vi "VI Tree.vi"   [LabVIEW 2025]
doc: "This is the instrument driver for the <INSTRUMENT NAME>. The VI Tree displays all the user-callable VIs of the instrument driver in an organized table."
panel:
  # "(c) 2025 RAMON TABOADA.  ALL RIGHTS RESERVED."
  # "SEE DIAGRAM\nFOR VI TREE."
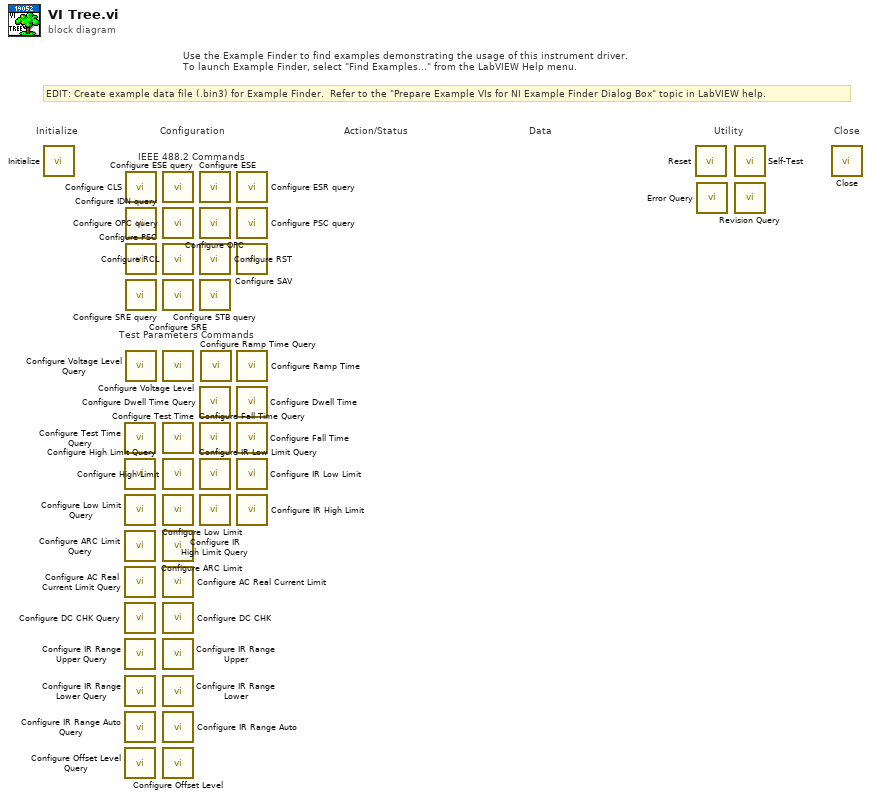
[diagram p0: block diagram]
diagram:
  # "Test Parameters Commands"
  # "IEEE 488.2 Commands"
  # "EDIT: Create example data file (.bin3) for Example Finder.  Refer to the \"Prepare Example VIs for NI Example Finder Dialog Box\" topic in LabVIEW help."
  # "Use the Example Finder to find examples demonstrating the usage of this instrument driver.\nTo launch Example Finder, select \"Find Examples...\" from the LabVIEW Help menu."
  # "Configuration"
  # "Utility"
  # "Data"
  # "Action/Status"
  # "Close"
  # "Initialize"
  n1 = call <instrlib>:"Initialize.vi"() -> ()  [unwired: 10 in, 2 out]
  n2 = call "Configure Test Time Query.vi"() -> ()  [unwired: 9 in, 3 out]
  n3 = call "Configure High Limit Query.vi"() -> ()  [unwired: 9 in, 3 out]
  n4 = call "Configure Low Limit Query.vi"() -> ()  [unwired: 9 in, 3 out]
  n5 = call "Configure ARC Limit Query.vi"() -> ()  [unwired: 9 in, 3 out]
  n6 = call "Configure AC Real Current Limit Query.vi"() -> ()  [unwired: 8 in, 3 out]
  n7 = call "Configure DC CHK Query.vi"() -> ()  [unwired: 10 in, 2 out]
  n8 = call "Configure IR Range Upper Query.vi"() -> ()  [unwired: 9 in, 3 out]
  n9 = call "Configure IR Range Lower Query.vi"() -> ()  [unwired: 9 in, 3 out]
  n10 = call "Configure IR Range Auto Query.vi"() -> ()  [unwired: 9 in, 3 out]
  n11 = call "Configure Offset Level Query.vi"() -> ()  [unwired: 10 in, 2 out]
  n12 = call "Configure CLS.vi"() -> ()  [unwired: 10 in, 2 out]
  n13 = call "Configure IDN query.vi"() -> ()  [unwired: 9 in, 3 out]
  n14 = call "Configure PSC.vi"() -> ()  [unwired: 10 in, 2 out]
  n15 = call "Configure SRE query.vi"() -> ()  [unwired: 9 in, 3 out]
  n16 = call "Configure Voltage Level Query.vi"() -> ()  [unwired: 9 in, 3 out]
  n17 = call "Configure ESE query.vi"() -> ()  [unwired: 9 in, 3 out]
  n18 = call "Configure OPC query.vi"() -> ()  [unwired: 9 in, 3 out]
  n19 = call "Configure RCL.vi"() -> ()  [unwired: 10 in, 2 out]
  n20 = call "Configure SRE.vi"() -> ()  [unwired: 10 in, 2 out]
  n21 = call "Configure Voltage Level.vi"() -> ()  [unwired: 10 in, 2 out]
  n22 = call "Configure Test Time.vi"() -> ()  [unwired: 10 in, 2 out]
  n23 = call "Configure High Limit.vi"() -> ()  [unwired: 10 in, 2 out]
  n24 = call "Configure Low Limit.vi"() -> ()  [unwired: 10 in, 2 out]
  n25 = call "Configure ARC Limit.vi"() -> ()  [unwired: 10 in, 2 out]
  n26 = call "Configure AC Real Current Limit.vi"() -> ()  [unwired: 9 in, 2 out]
  n27 = call "Configure DC CHK.vi"() -> ()  [unwired: 10 in, 2 out]
  n28 = call "Configure IR Range Upper.vi"() -> ()  [unwired: 10 in, 2 out]
  n29 = call "Configure IR Range Lower.vi"() -> ()  [unwired: 10 in, 2 out]
  n30 = call "Configure IR Range Auto.vi"() -> ()  [unwired: 10 in, 2 out]
  n31 = call "Configure Offset Level.vi"() -> ()  [unwired: 10 in, 2 out]
  n32 = call "Configure ESE.vi"() -> ()  [unwired: 10 in, 2 out]
  n33 = call "Configure OPC.vi"() -> ()  [unwired: 10 in, 2 out]
  n34 = call "Configure RST.vi"() -> ()  [unwired: 10 in, 2 out]
  n35 = call "Configure STB query.vi"() -> ()  [unwired: 9 in, 3 out]
  n36 = call "Configure Dwell Time Query.vi"() -> ()  [unwired: 9 in, 3 out]
  n37 = call "Configure Fall Time Query.vi"() -> ()  [unwired: 9 in, 3 out]
  n38 = call "Configure IR Low Limit Query.vi"() -> ()  [unwired: 9 in, 3 out]
  n39 = call "Configure IR High Limit Query.vi"() -> ()  [unwired: 9 in, 3 out]
  n40 = call "Configure Ramp Time Query.vi"() -> ()  [unwired: 9 in, 3 out]
  n41 = call "Configure ESR query.vi"() -> ()  [unwired: 9 in, 3 out]
  n42 = call "Configure PSC query.vi"() -> ()  [unwired: 9 in, 3 out]
  n43 = call "Configure SAV.vi"() -> ()  [unwired: 10 in, 2 out]
  n44 = call "Configure Ramp Time.vi"() -> ()  [unwired: 10 in, 2 out]
  n45 = call "Configure Dwell Time.vi"() -> ()  [unwired: 10 in, 2 out]
  n46 = call "Configure Fall Time.vi"() -> ()  [unwired: 10 in, 2 out]
  n47 = call "Configure IR Low Limit.vi"() -> ()  [unwired: 10 in, 2 out]
  n48 = call "Configure IR High Limit.vi"() -> ()  [unwired: 10 in, 2 out]
  n49 = call "Reset.vi"() -> ()  [unwired: 10 in, 2 out]
  n50 = call "Error Query.vi"() -> ()  [unwired: 8 in, 4 out]
  n51 = call "Self-Test.vi"() -> ()  [unwired: 8 in, 4 out]
  n52 = call "Revision Query.vi"() -> ()  [unwired: 8 in, 4 out]
  n53 = call "Close.vi"() -> ()  [unwired: 11 in, 1 out]
